vi "MainBaxterDemo.vi"() -> ()   [LabVIEW 2010]
uses:
  ROS/Code/_ROSDefinition.vi
  ROS/Code/SubVIs/BaxterSide.ctl
  ROS/Code/Slider.ctl
  ROS/Code/JointPositions.ctl
panel:
  out "Left Range Data":T1
  in  "Nod":bool
  in  "left gripper":u16(ring) items=["close"=0, "open"=100]
  in  "right gripper":u16(ring) items=["close"=0, "open"=100]
  in  "Parameters":T2 {"left_w2" scale=-180.0..180.0; "left_w1" scale=-180.0..180.0; "left_w0" scale=-180.0..180.0; "left_e1" scale=-180.0..180.0; "left_e0" scale=-180.0..180.0; "left_s1" scale=-180.0..180.0; "left_s0" scale=-180.0..180.0; "right_s1" scale=-180.0..180.0; "right_s0" scale=-180.0..180.0; "right_w2" scale=-180.0..180.0; "right_e1" scale=-180.0..180.0; "right_e0" scale=-180.0..180.0; "right_w0" scale=-180.0..180.0; "right_w1" scale=-180.0..180.0}
  out "Right Range Data":T1
  out "Joint States":T4(array[cluster])
  in  "disconnect head topic":bool
  in  "stop":bool
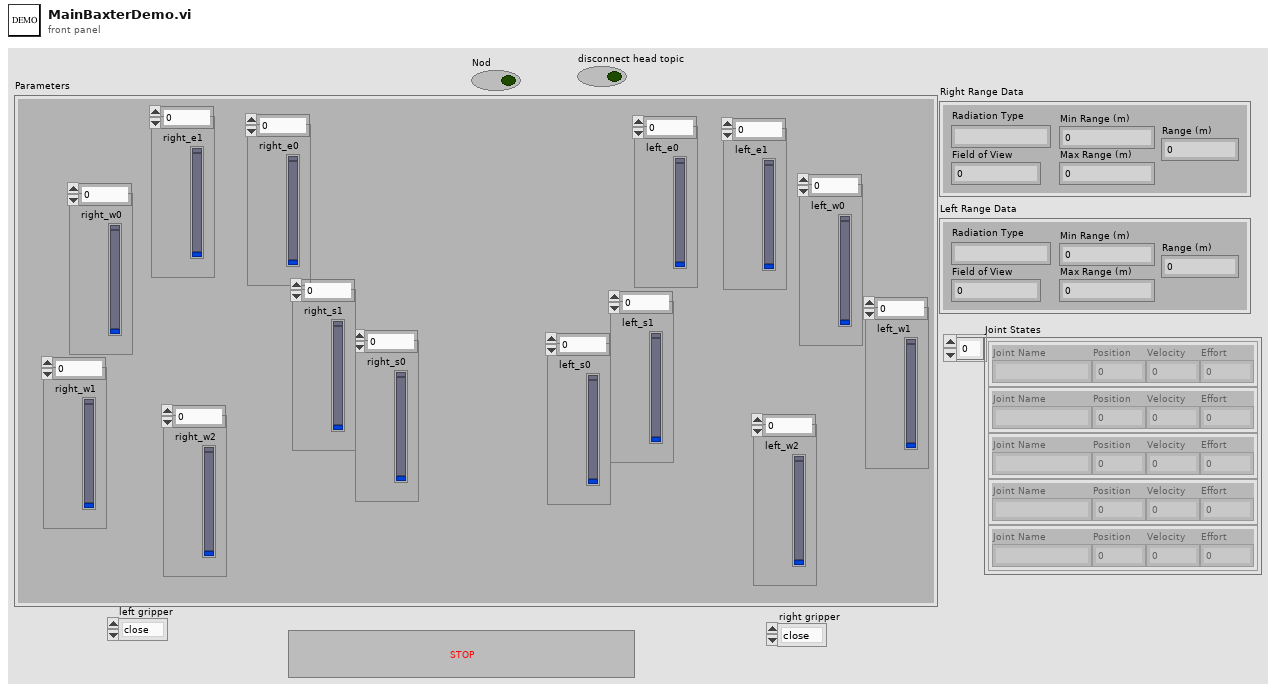
[diagram p1: front panel]
types:
  T1 = cluster{"Radiation Type":string, "Field of View":sgl, "Min Range (m)":sgl, "Max Range (m)":sgl, "Range (m)":sgl}
  T2 = typedef "JointPositions.ctl" = cluster{"left_e0":T3, "left_e1":T3, "left_s0":T3, "left_s1":T3, "left_w0":T3, "left_w1":T3, "left_w2":T3, "right_e0":T3, "right_e1":T3, "right_s0":T3, "right_s1":T3, "right_w0":T3, "right_w1":T3, "right_w2":T3}
  T3 = typedef "Slider.ctl" = dbl
  T4 = cluster{"Joint Name":string, "Position":dbl, "Velocity":dbl, "Effort":dbl}[]
  T5 = typedef "BaxterSide.ctl" = enum16{"left", "right"}
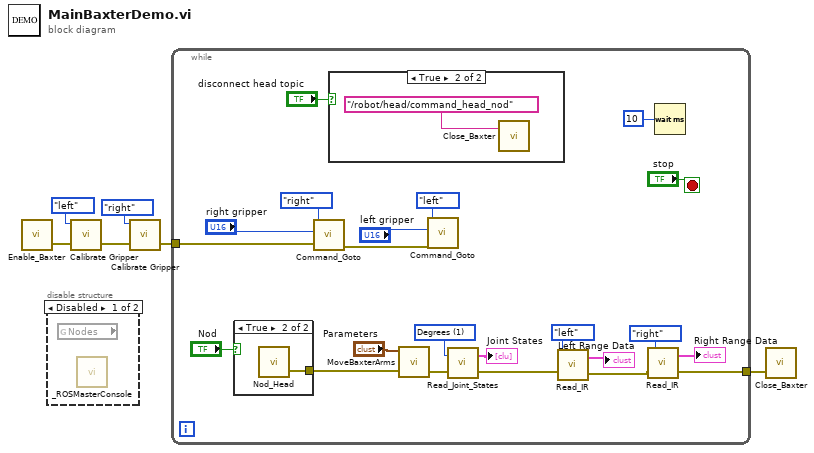
[diagram p0: block diagram]
diagram:
  n1 = call "Enable_Baxter.vi"() -> ("error out"=w5:errorcluster)  [unwired: 4 in]
  n2 = disable-structure shown="Disabled" {
    frame Disabled {
      n3 = global read "_ROSDefinition.vi" "Nodes"() -> ()  [unwired: 1 out]
      n4 = call "_ROSMasterConsole.vi"() -> ()  [unwired: 12 in]
    }
    frame Enabled {
    }
  }
  n5 = call "Calibrate Gripper.vi"("Side"=BaxterSide."left", "error in"=w5) -> ("error out"=w6:errorcluster)  [unwired: 4 in]
  n6 = call "Calibrate Gripper.vi"("Side"=BaxterSide."right", "error in"=w6) -> ("error out"=w4:errorcluster)  [unwired: 4 in]
  n7 = while {
    tunnel: [w25] -> w1
    tunnel: w4 -> [w20]
    stop <- "stop" stop-if-true
    w21 = u16 1 items=["Radians", "Degrees"] ("Units (Rad)")
    n8 = case shown="True" "Nod" {
      tunnel: [_ w30] -> w22
      frame False {
      }
      frame True {
        n9 = call "Nod_Head.vi"() -> ("error out"=w30:errorcluster)  [unwired: 4 in]
      }
    }
    n10 = call "Command_Goto.vi"("Side"=BaxterSide."right", "Desired Position"="right gripper", "error in"=w20) -> ("error out"=w18:errorcluster)  [unwired: 3 in]
    n11 = case shown="True" "disconnect head topic" {
      frame False {
      }
      frame True {
        n12 = call "Close_Baxter.vi"("topic"="/robot/head/command_head_nod") -> ()  [unwired: 3 in, 1 out]
      }
    }
    n13 = call "MoveBaxterArms.vi"("Parameters"="Parameters", "error in"=w22) -> ("error out"=w17:errorcluster)  [unwired: 4 in]
    n14 = call "Command_Goto.vi"("Side"=BaxterSide."left", "Desired Position"="left gripper", "error in"=w18) -> ()  [unwired: 3 in, 1 out]
    n15 = call "Read_Joint_States.vi"("error in"=w17, "Units (deg)"=w21) -> ("error out"=w10:errorcluster, "Joint States"=→"Joint States":T4)  [unwired: 1 in]
    n16 = call "Read_IR.vi"("error in"=w10, "Side"=BaxterSide."left") -> ("error out"=w9:errorcluster, "Range Data"=→"Left Range Data":T1)  [unwired: 1 in]
    n17 = call "Read_IR.vi"("error in"=w9, "Side"=BaxterSide."right") -> ("error out"=w25:errorcluster, "Range Data"=→"Right Range Data":T1)  [unwired: 1 in]
    n18 = Wait (ms)(milliseconds to wait=u32 10) -> ()  [unwired: 1 out]
  }
  n19 = call "Close_Baxter.vi"("error in"=w1) -> ()  [unwired: 3 in, 1 out]
